vi "NewTemplate.Start.vi"(5 "Autoshutdown? (T)":bool=TRUE, 8 "error in (no error)":errorcluster, 11 "NewTemplate in":refnum<class "SingleLoopTemplate.lvclass">) -> (0 "error out":errorcluster, 1 "StartupHandshake out":refnum<class "RQMHStartup.lvclass">, 2 "_TemplateModule":cluster{"Broadcasts":T1, "Broadcasts":T2}, 3 "NewTemplate out":refnum<class "SingleLoopTemplate.lvclass">)   [LabVIEW 2025, in "SingleLoopTemplate.lvclass"]
uses:
  SingleLoopTemplate.lvclass
  SingleLoopTemplate.lvclass/SingleLoopTemplate.ctl
  Stopped.ctl
  Broadcast Events--cluster.ctl
  RQMHCore/Shared/Died.ctl
  RQMHCore/ModuleCore/StandardBroadcasts.ctl
  RQMHCore/ModuleCore/Started.ctl
  RQMHCore/Startup/RQMHStartup.lvclass
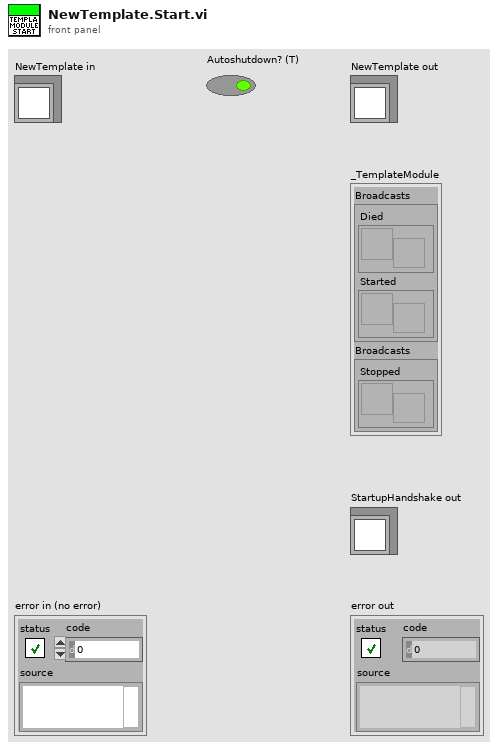
[diagram p1: front panel]
types:
  T1 = typedef "RQMHModule.lvclass/StandardBroadcasts.ctl" = cluster{"Died":refnum<user-event>, "Started":refnum<user-event>}
  T2 = typedef "SingleLoopTemplate.lvclass/Broadcast Events--cluster.ctl" = cluster{"Stopped":refnum<user-event>}
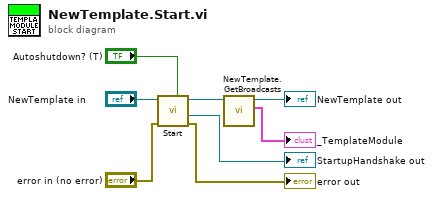
[diagram p0: block diagram]
diagram:
  n1 = call "Start.vi"("Autoshutdown? (T)"="Autoshutdown? (T)", "error in (no error)"="error in (no error)", "JQMHCore in"="NewTemplate in") -> ("error out"=→"error out":errorcluster, "StartupHandshake out"=→"StartupHandshake out":refnum<class "RQMHStartup.lvclass">, "JQMHCore out"=w4:refnum<class "SingleLoopTemplate.lvclass">)  [unwired: 6 in]
  n2 = call "NewTemplate.GetBroadcasts.vi"("NewTemplate in"=w4) -> ("TemplateModule"=→"_TemplateModule":cluster{"Broadcasts":T1, "Broadcasts":T2}, "NewTemplate out"=→"NewTemplate out":refnum<class "SingleLoopTemplate.lvclass">)  [unwired: 9 in]
